vi "API_Init.vi"(1 "API Option":enum16{"None", "Blocking", "Wait for Input"}(ring), 2 "API Mode":T1(ring)=enum."Instantaneous", 3 "VI Path":path, 4 "Argument List In":string[](array[string])) -> (0 "Argument List Out":string[](array[string]))   [LabVIEW 2011]
doc: "This VI opens a reference to the calling API VI via the \"VI Path\" parameter, initializes the \"Argument List\" if necessary, then updates the calling API VI's front panel controls and indicators according to the values stored in the \"Argument List\". For more information on the \"API Mode\" parameter, refer to Set_API_Mode.vi. This VI also initializes the window mode of the API VI."
panel:
  out "Error Out":errorcluster
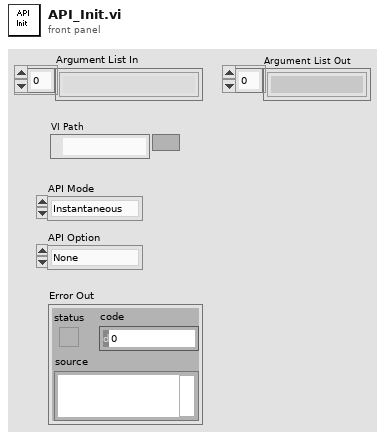
[diagram p1: front panel]
types:
  T1 = enum16{"Discrete", "Continuous", "Instantaneous", "Finite"}
  T2 = enum32{"Invalid", "Default", "Floating", "Floating/Auto-Hide", "Modal"}
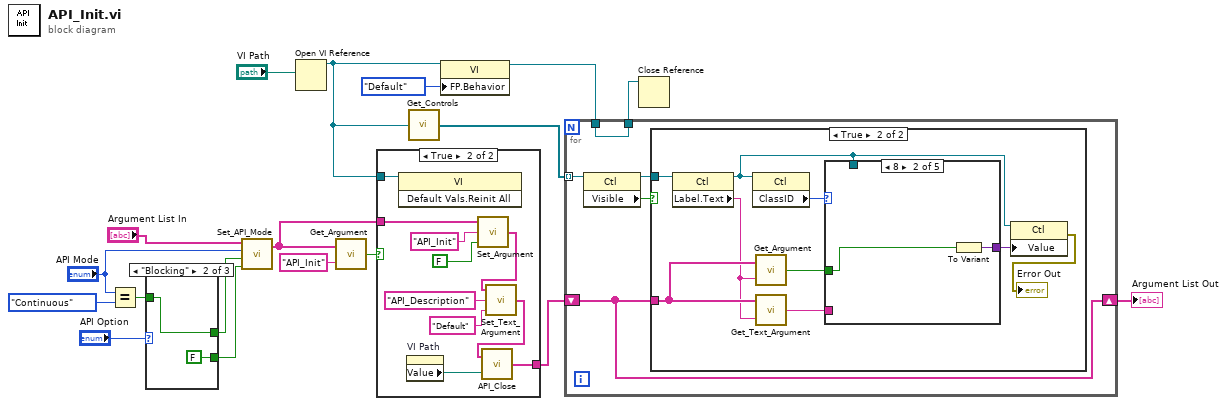
[diagram p0: block diagram]
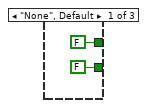
[diagram p2: hidden frame]
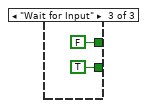
[diagram p3: hidden frame]
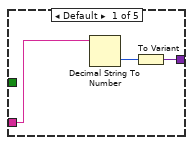
[diagram p5: hidden frame]
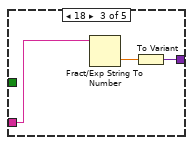
[diagram p6: hidden frame]
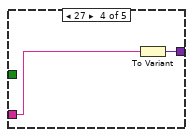
[diagram p7: hidden frame]
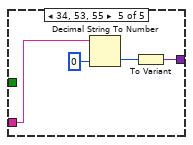
[diagram p8: hidden frame]
diagram:
  n1 = Equal?(x="API Mode", y=T1."Continuous" ("API Mode")) -> (x = y?=w6:bool)
  n2 = case shown="\"Blocking\"" "API Option" {
    tunnel: [FALSE w21 FALSE] -> w9
    tunnel: [FALSE FALSE TRUE] -> w8
    tunnel: w6 -> [_ w21 _]
    frame "None", Default {
    }
    frame "Blocking" {
    }
    frame "Wait for Input" {
    }
  }
  n3 = call "Set_API_Mode.vi"("Wait for Input"=w8, "API Blocking"=w9, "API Mode"="API Mode", "Argument List In"="Argument List In") -> ("Argument List Out"=w15:string[])  [unwired: 1 in]
  n4 = Open VI Reference(vi path="VI Path") -> (vi reference=w2:refnum<vi>)  [unwired: 5 in, 1 out]
  n5 = call "Get_Argument.vi"("Argument"="API_Init", "Argument List"=w15) -> ("Enabled"=w17:bool)
  n6 = case shown="True" w17 {
    tunnel: w15 -> [w25 w35]
    tunnel: [w25 w26] -> w16
    tunnel: w2 -> [_ w29]
    frame False {
    }
    frame True {
      n7 = invoke class="VI" method="Default Vals.Reinit All"(reference=w29) -> ()  [unwired: 2 in, 3 out]
      n8 = property on="VI Path" class="Path"() -> ("Value"=w27:path)  [unwired: 2 in, 2 out]
      n9 = call "Set_Argument.vi"("Enable"=FALSE, "Argument"="API_Init", "Argument List In"=w35) -> ("Argument List Out"=w32:string[])
      n10 = call "Set_Text_Argument.vi"("Text"="Default", "Argument"="API_Description", "Argument List In"=w32) -> ("Argument List Out"=w28:string[])
      n11 = call "API_Close.vi"("VI Path"=w27, "Argument List In"=w28) -> ("Argument List Out"=w26:string[])
    }
  }
  n12 = call "Get_Controls.vi"("VI Reference"=w2) -> ("Controls"=w5:refnum<vi>[])
  n13 = property class="VI"(reference=w2, "FP.Behavior"=T2."Default" ("Front Panel Window:Behavior")) -> (reference out=w4:refnum<vi>)  [unwired: 1 in, 1 out]
  n14 = for {
    tunnel: w5 -> [w39] mode=indexing
    shift-right: [w40] -> w13
    shift-left: w16 -> [w40]
    tunnel: w4 -> [w36]
    tunnel: [w36] -> w3
    n15 = property class="Ctl"(reference=w39) -> (reference out=w38:refnum<vi>, "Visible"=w37:bool)  [unwired: 1 in, 1 out]
    n16 = case shown="True" w37 {
      tunnel: w40 -> [_ w45]
      tunnel: w38 -> [_ w42]
      frame False {
      }
      frame True {
        n17 = property class="Ctl"(reference=w42) -> (reference out=w41:refnum<vi>, "Label.Text"=w44:string)  [unwired: 1 in, 1 out]
        n18 = property class="Ctl"(reference=w41) -> ("ClassID"=w49:u32)  [unwired: 1 in, 2 out]
        n19 = call "Get_Argument.vi"("Argument"=w44, "Argument List"=w45) -> ("Enabled"=w43:bool)
        n20 = call "Get_Text_Argument.vi"("Argument"=w44, "Argument List"=w45) -> ("Text"=w48:string)
        n21 = case shown="8" w49 {
          tunnel: w48 -> [w52 _ w57 w58 w63]
          tunnel: [w51 w54 w56 w59 w62] -> w47
          tunnel: w43 -> [_ w53 _ _ _]
          tunnel: w41 -> [_ _ _ _ _]
          frame Default {
            n22 = Decimal String To Number(string=w52) -> (number=w50:i32)  [unwired: 2 in, 1 out]
            n23 = To Variant(anything=w50) -> (Variant=w51:variant)
          }
          frame 8 {
            n24 = To Variant(anything=w53) -> (Variant=w54:variant)
          }
          frame 18 {
            n25 = Fract/Exp String To Number(string=w57) -> (number=w55:dbl)  [unwired: 3 in, 1 out]
            n26 = To Variant(anything=w55) -> (Variant=w56:variant)
          }
          frame 27 {
            n27 = To Variant(anything=w58) -> (Variant=w59:variant)
          }
          frame 34, 53, 55 {
            n28 = Decimal String To Number(string=w63, default (0L)=u16 0 ("default (0 I32)")) -> (number=w61:u16)  [unwired: 1 in, 1 out]
            n29 = To Variant(anything=w61) -> (Variant=w62:variant)
          }
        }
        n30 = property class="Ctl"(reference=w41, "Value"=w47) -> (error out=→"Error Out":errorcluster)  [unwired: 1 in, 1 out]
      }
    }
  }
  "Argument List Out" <- w13
  n31 = Close Reference(reference=w3) -> ()  [unwired: 1 in, 1 out]
